vi "Counter - Read Pulse Width and Frequency (Finite).vi"() -> ()   [LabVIEW 2017]
doc: "本范例演示对有限数量的采样执行周期、频率、脉冲宽度，脉冲宽度，或两边沿间隔等类型测量的方法。\n\n本范例采用隐式定时，即输入信号的每个周期采集一个采样。\n\n关于将信号连接至DAQ设备的方法，可参考设备文档。"
uses:
  <vilib>/Utility/error.llb/DialogType.ctl
  <vilib>/DAQmx/read.llb/DAQmx Read (Counter 1D DBL 1Chan NSamp).vi
  <vilib>/DAQmx/create/channels.llb/DAQmx Create Channel (CI-Period).vi
  <vilib>/DAQmx/create/channels.llb/DAQmx Create Channel (CI-Frequency).vi
  <vilib>/DAQmx/create/channels.llb/DAQmx Create Channel (CI-Pulse Width).vi
  <vilib>/DAQmx/create/channels.llb/DAQmx Create Channel (CI-Two Edge Separation).vi
  <vilib>/DAQmx/configure/timing.llb/DAQmx Timing (Implicit).vi
  <vilib>/DAQmx/miscellaneous.llb/DAQmx Fill In Error Info.vi
  <resource>/objmgr/daqmx.rc
panel:
  out "数据":dbl[](array[numeric])
  in  "计数器输入类型":T1(tab)
  in  "周期输入接线端":tag="/Dev1/PFI9"
  in  "最大周期":dbl=0.1 format="%0.6f"
  in  "最小周期":dbl=1e-06 format="%0.6f"
  in  "最小频率":dbl=2.0 format="%0.6f"
  in  "最大频率":dbl=100.0 format="%0.6f"
  in  "频率输入接线端":tag="/Dev1/PFI9"
  in  "脉冲宽度输入接线端":tag="/Dev1/PFI9"
  in  "最小脉冲宽度":dbl=1e-06 format="%0.6f"
  in  "最大脉冲宽度":dbl=0.1 format="%0.6f"
  in  "第二个输入信号":tag="/Dev1/PFI9"
  in  "第一个输入接线端":tag="/Dev1/PFI10"
  in  "最小间隔时间":dbl=1e-06 format="%0.6f"
  in  "最大间隔时间":dbl=0.1 format="%0.6f"
  in  "采样数":i32=1000
  in  "计数器":tag="Dev1/ctr0"
  # "通道设置"
  # "采集数据"
  # "定时设置"
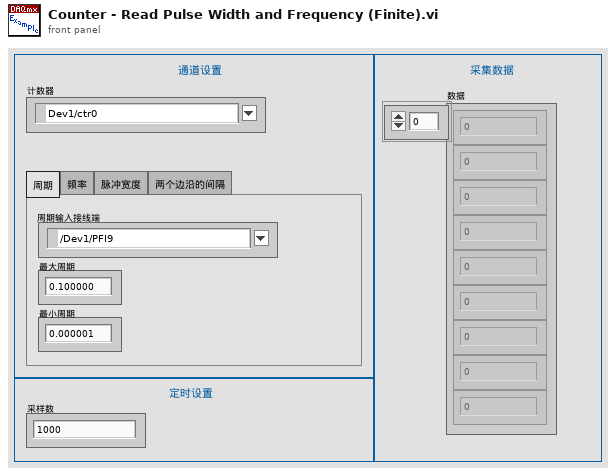
[diagram p1: front panel]
types:
  T1 = enum32{"Period", "Frequency", "Pulse Width", "2 Edge Separation"}
  T2 = typedef "DialogType.ctl" = u16
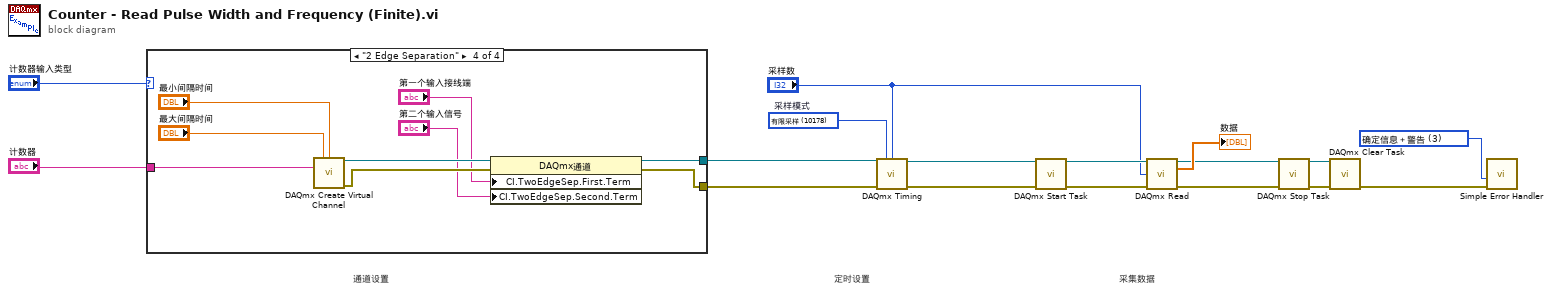
[diagram p0: block diagram]
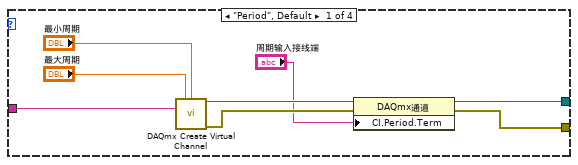
[diagram p2: hidden frame]
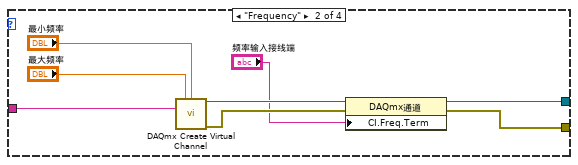
[diagram p3: hidden frame]
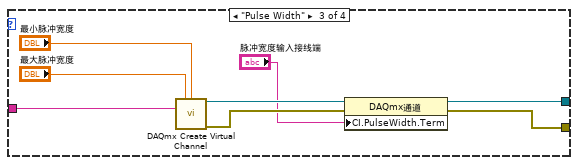
[diagram p4: hidden frame]
diagram:
  w1 = T2 3 items=["无对话框", "确定信息", "继续或停止信息", "确定信息＋警告", "继续/停止＋警告"] ("对话框类型（确定信息：1）")
  w17 = 10178 items=["有限采样"=10178, "连续采样"=10123, "硬件定时单点"=12522]  # 采样模式
  # "采集数据"
  # "定时设置"
  # "通道设置"
  n1 = case shown="\"2 Edge Separation\"" "计数器输入类型" {
    tunnel: [w23 w31 w39 w48] -> w16
    tunnel: [w24 w32 w40 w49] -> w15
    tunnel: "计数器" -> [w25 w33 w41 w50]
    frame "Period", Default {
      n2 = call-poly <vilib>:"DAQmx Create Virtual Channel.vi"("maximum value"="最大周期", "minimum value"="最小周期", "counter"=w25) -> ("task out"=w22:refnum<k21>, "error out"=w21:errorcluster)  [unwired: 11 in]
      n3 = property class="DAQmx通道"(reference=w22, error in=w21, "CI.Period.Term"="周期输入接线端") -> (reference out=w24:refnum<k21>, error out=w23:errorcluster)
    }
    frame "Frequency" {
      n4 = call-poly <vilib>:"DAQmx Create Virtual Channel.vi"("maximum value"="最大频率", "minimum value"="最小频率", "counter"=w33) -> ("task out"=w30:refnum<k21>, "error out"=w29:errorcluster)  [unwired: 11 in]
      n5 = property class="DAQmx通道"(reference=w30, error in=w29, "CI.Freq.Term"="频率输入接线端") -> (reference out=w32:refnum<k21>, error out=w31:errorcluster)
    }
    frame "Pulse Width" {
      n6 = call-poly <vilib>:"DAQmx Create Virtual Channel.vi"("maximum value"="最大脉冲宽度", "minimum value"="最小脉冲宽度", "counter"=w41) -> ("task out"=w38:refnum<k21>, "error out"=w37:errorcluster)  [unwired: 11 in]
      n7 = property class="DAQmx通道"(reference=w38, error in=w37, "CI.PulseWidth.Term"="脉冲宽度输入接线端") -> (reference out=w40:refnum<k21>, error out=w39:errorcluster)
    }
    frame "2 Edge Separation" {
      n8 = call-poly <vilib>:"DAQmx Create Virtual Channel.vi"("maximum value"="最大间隔时间", "minimum value"="最小间隔时间", "counter"=w50) -> ("task out"=w47:refnum<k21>, "error out"=w46:errorcluster)  [unwired: 11 in]
      n9 = property class="DAQmx通道"(reference=w47, error in=w46, "CI.TwoEdgeSep.First.Term"="第一个输入接线端", "CI.TwoEdgeSep.Second.Term"="第二个输入信号") -> (reference out=w49:refnum<k21>, error out=w48:errorcluster)
    }
  }
  n10 = call-poly <vilib>:"DAQmx Timing.vi"("task/channels in"=w15, "sample mode"=w17, "samples per channel"="采样数", "error in"=w16) -> ("task out"=w9:refnum<k21>, "error out"=w8:errorcluster)  [unwired: 10 in]
  n11 = call <vilib>:"DAQmx Start Task.vi"("task/channels in"=w9, "error in"=w8) -> ("task out"=w14:refnum<k21>, "error out"=w13:errorcluster)  [unwired: 12 in]
  n12 = call-poly <vilib>:"DAQmx Read.vi"("task/channels in"=w14, "number of samples per channel"="采样数", "error in"=w13) -> ("task out"=w3:refnum<k21>, "data"=→"数据":dbl[], "error out"=w2:errorcluster)  [unwired: 10 in]
  n13 = call <vilib>:"DAQmx Stop Task.vi"("task/channels in"=w3, "error in"=w2) -> ("task out"=w5:refnum<k21>, "error out"=w4:errorcluster)  [unwired: 12 in]
  n14 = call <vilib>:"DAQmx Clear Task.vi"("task in"=w5, "error in"=w4) -> ("error out"=w12:errorcluster)  [unwired: 13 in]
  n15 = call <vilib>:"Simple Error Handler.vi"("type of dialog (OK msg:1)"=w1, "error in (no error)"=w12) -> ()  [unwired: 3 in, 5 out]
